vi "FileRW_CalConst.vi"(7 "RW":enum16{"Read", "Write"}(ring), 8 "error in":errorcluster, 10 "Cal Const IN":T1(array[cluster]) {"PSlope" format="%#.13f"; "NSlope" format="%#.13f"; "AvgSlope" format="%#.13f"; "Center" format="%#.13f"; "Offset" format="%#.13f"}, 11 "IP Address":string) -> (0 "error out":errorcluster, 2 "Cal Const OUT":T1(array[cluster]) {"PSlope" format="%#.13f"; "NSlope" format="%#.13f"; "AvgSlope" format="%#.13f"; "Center" format="%#.13f"; "Offset" format="%#.13f"})   [LabVIEW 2015]
uses:
  Anemometry/Anemometry Sub Vis/File/Setup_Filetype.ctl
panel:
  in  "Tab Control":enum32{"Input", "Output"}(tab)
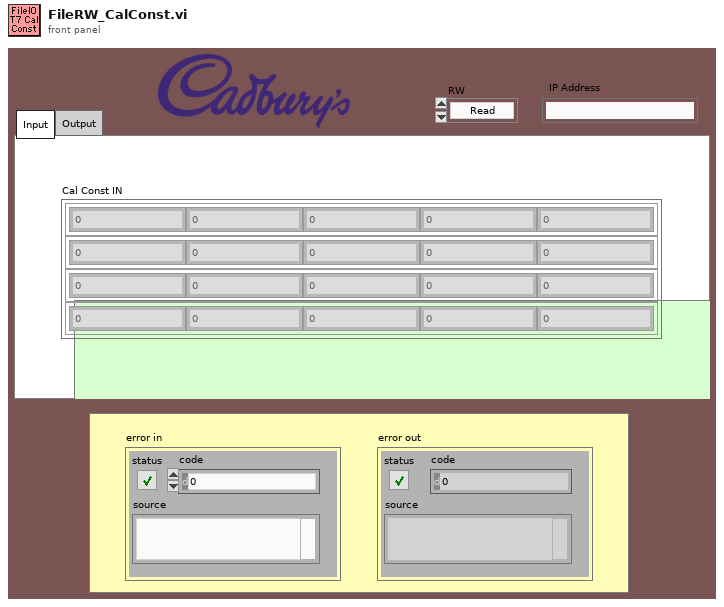
[diagram p1: front panel]
types:
  T1 = cluster{"PSlope":dbl, "NSlope":dbl, "AvgSlope":dbl, "Center":dbl, "Offset":dbl}[]
  T2 = typedef "Setup_Filetype.ctl" = enum16{"Measurement Setups", "Calibration Setups", "General", "Results File Plotter Setups", "Speed Calib Tweaks"}
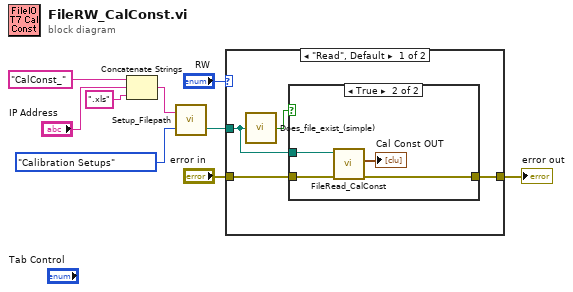
[diagram p0: block diagram]
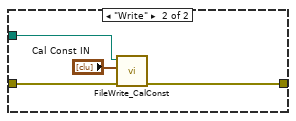
[diagram p3: hidden frame]
diagram:
  n1 = Concatenate Strings("CalConst_" ("Dashboard Config Filename"), "IP Address", ".xls") -> (w3:string)
  n2 = call "Setup_Filepath.vi"("Setup File Type"=Setup_Filetype."Calibration Setups", "Filename in"=w3) -> ("Filename Out"=w7:path)  [unwired: 1 out]
  n3 = case shown="\"Read\", Default" "RW" {
    tunnel: w7 -> [w10 w20]
    tunnel: [w13 w21] -> w1
    tunnel: "error in" -> [w12 w22]
    frame "Read", Default {
      n4 = call "Does_file_exist_(simple).vi"("Pathname"=w10) -> ("exists?"=w11:bool)
      n5 = case shown="True" w11 {
        tunnel: [w14 w17] -> w13
        tunnel: w12 -> [w14 w18]
        tunnel: w10 -> [_ w16]
        frame False {
        }
        frame True {
          n6 = call "FileRead_CalConst.vi"("error in"=w18, "file path (use dialog)"=w16) -> ("error out"=w17:errorcluster, "Calibration Constants"=→"Cal Const OUT":T1)  [unwired: 8 in]
        }
      }
    }
    frame "Write" {
      n7 = call "FileWrite_CalConst.vi"("error in"=w22, "Calibration Constants"="Cal Const IN", "file path (use dialog)"=w20) -> ("error out"=w21:errorcluster)  [unwired: 8 in]
    }
  }
  "error out" <- w1
